vi "Menu Act.vi"(10 "LayoutMap":map{string, T1}(c390), 11 "Menu in":refnum<k9>) -> ()   [LabVIEW 2020, in "MDI ViewManager.lvlib"]
uses:
  MDI ViewManager.lvlib
  Typedef/Layout.ctl
  <vilib>/Utility/miscctls.llb/LVPointTypeDef.ctl
  <vilib>/Utility/miscctls.llb/LVBoundsTypeDef.ctl
  <vilib>/Utility/miscctls.llb/LVPositionTypeDef.ctl
  <vilib>/Utility/miscctls.llb/LVRectTypeDef.ctl
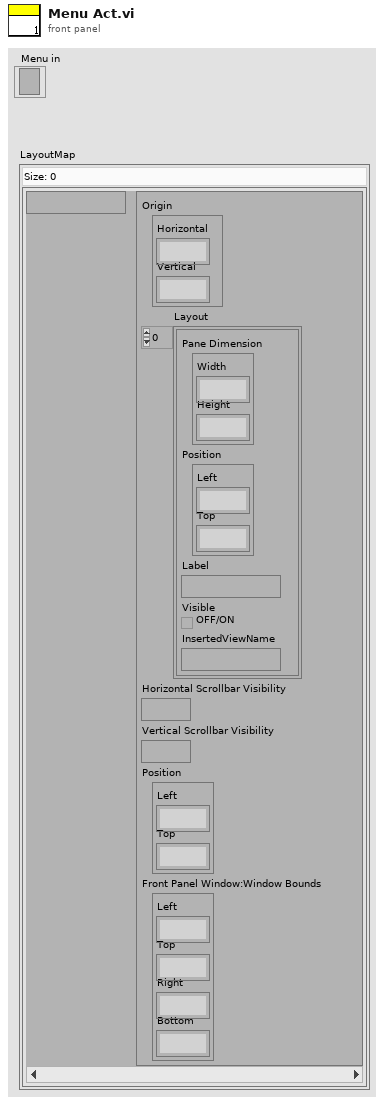
[diagram p1: front panel]
types:
  T1 = typedef "MDI ViewManager.lvlib/Layout.ctl" = cluster{"Origin":T2, "Layout":cluster{"Pane Dimension":T3, "Position":T4, "Label":string, "Visible":bool, "InsertedViewName":string}[], "Horizontal Scrollbar Visibility":enum16{"Always On", "Always Off", "Off While Running"}, "Vertical Scrollbar Visibility":enum16{"Always On", "Always Off", "Off While Running"}, "Position":T4, "Rect":T5}
  T2 = typedef "LVPointTypeDef.ctl" = cluster{"Horizontal":i16, "Vertical":i16}
  T3 = typedef "LVBoundsTypeDef.ctl" = cluster{"Width":u32, "Height":u32}
  T4 = typedef "LVPositionTypeDef.ctl" = cluster{"Left":i32, "Top":i32}
  T5 = typedef "LVRectTypeDef.ctl" = cluster{"Left":i16, "Top":i16, "Right":i16, "Bottom":i16}
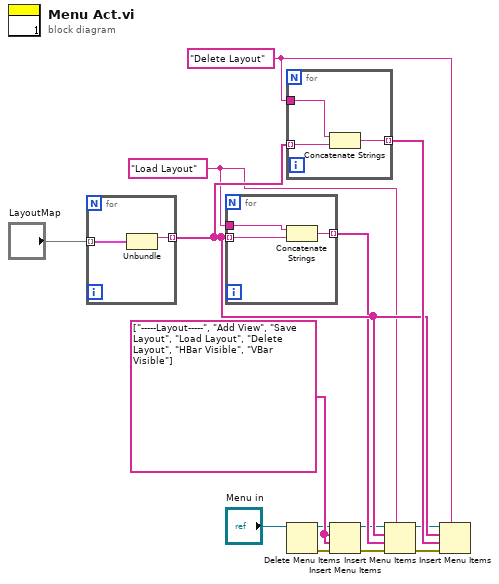
[diagram p0: block diagram]
diagram:
  w12 = "Delete Layout"
  w10 = "Load Layout"
  w3 = string[] ["-----Layout-----", "Add View", "Save Layout", "Load Layout", "Delete Layout", "HBar Visible", "VBar Visible"] ("item names")
  n1 = for {
    tunnel: "LayoutMap" -> [w16] mode=indexing
    tunnel: [w15] -> w13 mode=indexing
    n2 = Unbundle(w16) -> (w15:string)  [unwired: 1 out]
  }
  n3 = for {
    tunnel: w13 -> [w19] mode=indexing
    tunnel: w10 -> [w18]
    tunnel: [w17] -> w11 mode=indexing
    n4 = Concatenate Strings(w18, w19) -> (w17:string)
  }
  n5 = for {
    tunnel: w13 -> [w22] mode=indexing
    tunnel: w12 -> [w21]
    tunnel: [w20] -> w14 mode=indexing
    n6 = Concatenate Strings(w21, w22) -> (w20:string)
  }
  n7 = Delete Menu Items(9:"Menu in") -> (0:w1:errorcluster, 3:w2:refnum<k9>)  [unwired: 3 in]
  n8 = Insert Menu Items(6:w1, 7:w3, 8:w3, 9:w2) -> (0:w6:errorcluster, 3:w7:refnum<k9>)  [unwired: 2 in, 1 out]
  n9 = Insert Menu Items(5:w10, 6:w6, 7:w11, 8:w13, 9:w7) -> (0:w9:errorcluster, 3:w8:refnum<k9>)  [unwired: 1 in, 1 out]
  n10 = Insert Menu Items(5:w12, 6:w9, 7:w14, 8:w13, 9:w8) -> ()  [unwired: 1 in, 3 out]
